vi "Com Write.vi"(8 "错误输入（无错误）":errorcluster, 10 "Wbuff":string, 11 "VISA In":refnum<visa-resource-name>) -> (0 "错误输出":errorcluster, 3 "VISA Out":refnum<visa-resource-name>)   [LabVIEW 2015]
uses:
  <vilib>/Instr/_visa.llb/VISA Flush IO Buffer Mask.ctl
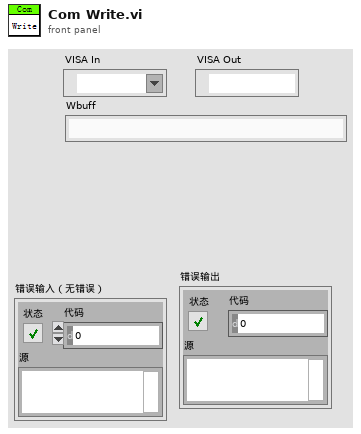
[diagram p1: front panel]
types:
  T1 = typedef "VISA Flush IO Buffer Mask.ctl" = u16
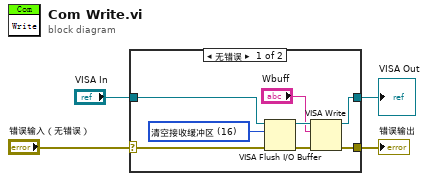
[diagram p0: block diagram]
diagram:
  n1 = case shown="无错误" "错误输入（无错误）" {
    selector: "错误输入（无错误）" -> [w6 w14]
    tunnel: "VISA In" -> [w12 w13]
    tunnel: [w7 w14] -> w3
    tunnel: [w5 w13] -> w1
    frame No Error {
      w10 = T1 16 items=["清空接收缓冲区"=16, "向设备写入传输缓冲区"=32, "清空接收缓冲区（无I/O）"=64, "清空传输缓冲区"=128] ("Mask")
      n2 = VISA Flush I/O Buffer(VISA resource name=w12, mask (16)=w10, error in (no error)=w6) -> (VISA resource name out=w11:refnum<visa-resource-name>, error out=w9:errorcluster)
      n3 = VISA Write(VISA resource name=w11, write buffer="Wbuff", error in (no error)=w9) -> (VISA resource name out=w5:refnum<visa-resource-name>, error out=w7:errorcluster)  [unwired: 1 out]
    }
    frame Error {
    }
  }
  "错误输出" <- w3
  "VISA Out" <- w1
